vi "CAM_file_swap.vi"(8 "error in":errorcluster, 10 "DUT":string="1", 11 "Barcode":string) -> (0 "error out":errorcluster, 1 "Ref_img_path":path, 2 "DTU_Conf":string, 3 "image path":path)   [LabVIEW 2024, in "Keyence_VS150.lvlib"]
uses:
  Keyence_VS150.lvlib
  Launcher/Launcher_DTU.lvlib
panel:
  out "result string":string
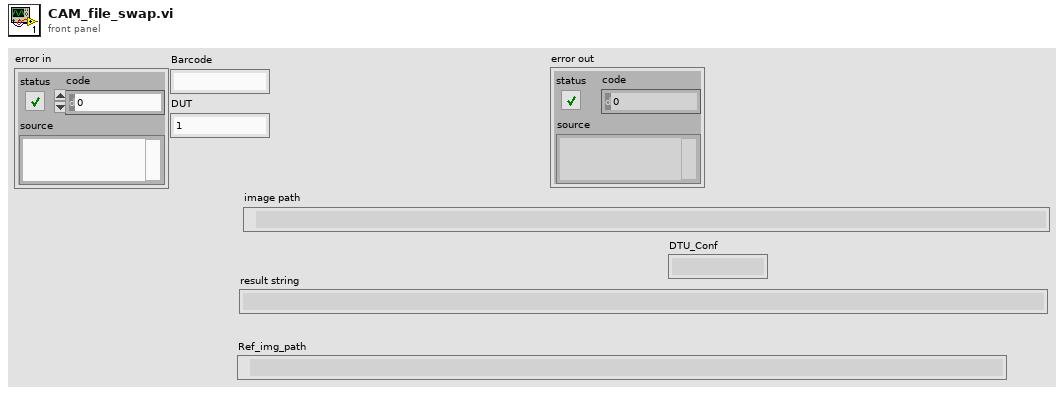
[diagram p1: front panel]
types:
  T1 = enum16{"Read", "Write", "All_sections", "All_values", "Remove key&section"}
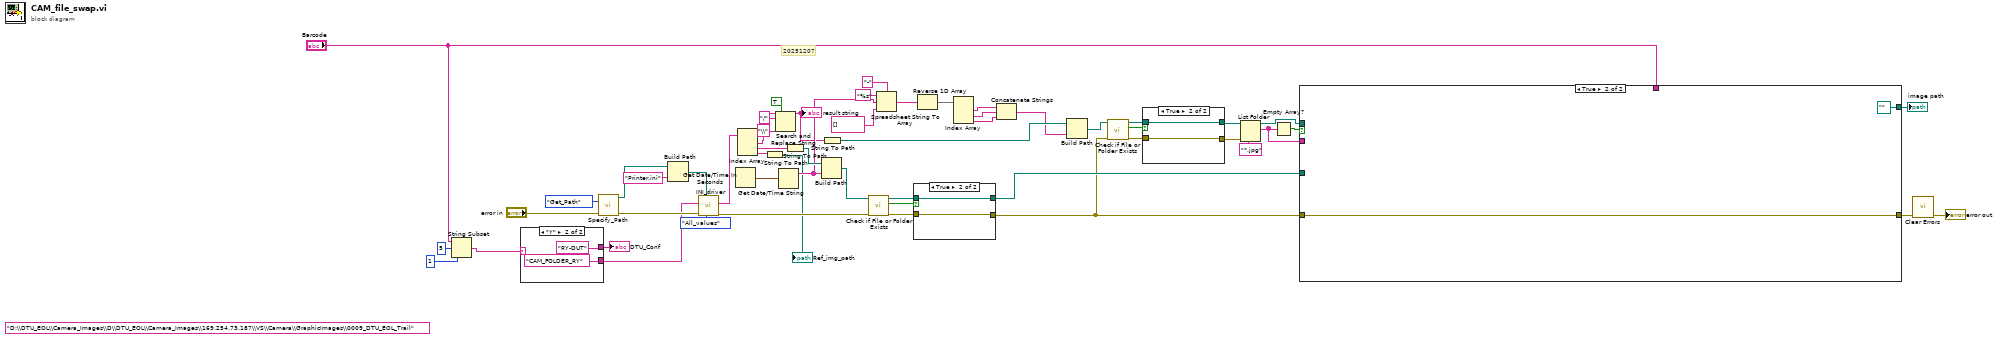
[diagram p0: block diagram]
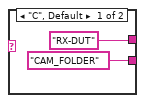
[diagram p2: hidden frame]
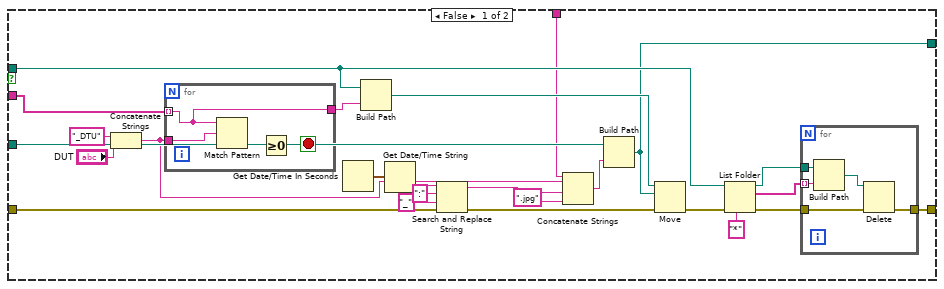
[diagram p3: hidden frame]
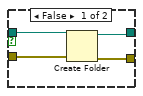
[diagram p4: hidden frame]
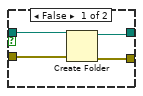
[diagram p5: hidden frame]
diagram:
  (unwired) "D:\\DTU_EOL\\Camera_Images\\D\\DTU_EOL\\Camera_Images\\169.254.73.187\\VS\\Camera\\GraphicImages\\0009_DTU_EOL_Trail"
  # "20251207"
  n1 = String Subset(string="Barcode", offset (0)=5, length (rest)=1 ("length (rest)")) -> (substring=w7:string)
  n2 = case shown="\"Y\"" w7 {
    tunnel: ["CAM_FOLDER" ("Section") "CAM_FOLDER_RY" ("Section")] -> w6
    tunnel: ["RX-DUT" "RY-DUT"] -> w3
    frame "C", Default {
    }
    frame "Y" {
    }
  }
  "DTU_Conf" <- w3
  n3 = call "Specify_Path.vi"("Path_Enum"=enum16{"Find_Path", "Get_Path"}."Get_Path", "error in (no error)"="error in") -> ("Configurations"=w52:path, "error out"=w53:errorcluster)  [unwired: 6 in, 6 out]
  n4 = Build Path(base path=w52, name or relative path="Printer.ini") -> (appended path=w50:path)
  n5 = call "INI_driver.vi"("Enum"=T1."All_values", "instrument file path"=w50, "error in (no error)"=w53, "Section"=w6) -> ("error out"=w45:errorcluster, "Values out"=w48:string[])  [unwired: 4 in, 2 out]
  n6 = Get Date/Time In Seconds() -> (seconds since 1Jan1904=w47:timestamp)
  n7 = Index Array(array=w48) -> (element #1=w14:string, element #2=w41:string, element #3=w2:string)  [unwired: 3 in]
  n8 = String To Path(string=w2) -> (path=→"Ref_img_path":path)
  n9 = Search and Replace String(replace all?=TRUE ("replace all? (F)"), input string=w14, search string="/", replace string="\\" ("replace string (\"\")")) -> (result string=w11:string)  [unwired: 4 in, 3 out]
  "result string" <- w11
  n10 = Get Date/Time String(seconds (now)=w47) -> (date string=w29:string)  [unwired: 2 in, 1 out]
  n11 = String To Path(string=w41) -> (path=w40:path)
  n12 = Build Path(base path=w40, name or relative path=w29) -> (appended path=w46:path)
  n13 = String To Path(string=w11) -> (path=w28:path)
  n14 = call <vilib>:"Check if File or Folder Exists.vi"("error in (no error)"=w45, "path"=w46) -> ("error out"=w42:errorcluster, "file or folder exists?"=w44:bool, "dup path"=w43:path)  [unwired: 7 in]
  n15 = Spreadsheet String To Array(delimiter (Tab)="-", format string="%s", spreadsheet string=w29, array type (2D Dbl)=string[] []) -> (array=w34:string[])
  n16 = case shown="True" w44 {
    tunnel: w43 -> [w62 w64]
    tunnel: w42 -> [w63 w65]
    tunnel: [w61 w65] -> w22
    tunnel: [w60 w64] -> w39
    frame False {
      n17 = Create Folder(path (use dialog)=w62, error in=w63) -> (created path=w60:path, error out=w61:errorcluster)  [unwired: 1 in, 1 out]
    }
    frame True {
    }
  }
  n18 = Reverse 1D Array(array=w34) -> (reversed array=w33:string[])
  n19 = Index Array(array=w33) -> (element #1=w32:string, element #2=w31:string, element #3=w30:string)  [unwired: 3 in]
  n20 = Concatenate Strings(w32, w31, w30) -> (w27:string)
  n21 = Build Path(base path=w28, name or relative path=w27) -> (appended path=w23:path)
  n22 = call <vilib>:"Check if File or Folder Exists.vi"("error in (no error)"=w22, "path"=w23) -> ("error out"=w26:errorcluster, "file or folder exists?"=w24:bool, "dup path"=w25:path)  [unwired: 7 in]
  n23 = case shown="True" w24 {
    tunnel: w25 -> [w68 w70]
    tunnel: w26 -> [w69 w71]
    tunnel: [w67 w71] -> w21
    tunnel: [w66 w70] -> w20
    frame False {
      n24 = Create Folder(path (use dialog)=w68, error in=w69) -> (created path=w66:path, error out=w67:errorcluster)  [unwired: 1 in, 1 out]
    }
    frame True {
    }
  }
  n25 = List Folder(path=w20, pattern="*.jpg", error in=w21) -> (path out=w17:path, filenames=w16:string[])  [unwired: 1 in, 2 out]
  n26 = Empty Array?(array=w16) -> (empty?=w18:bool)
  n27 = case shown="True" w18 {
    tunnel: w39 -> [w95 _]
    tunnel: [w78 w106] -> w38
    tunnel: w22 -> [w87 w106]
    tunnel: w17 -> [w74 _]
    tunnel: w16 -> [w84 _]
    tunnel: "Barcode" -> [w73 _]
    tunnel: [w72 path "" ("appended path")] -> w4
    frame False {
      n28 = Concatenate Strings("_DTU", "DUT") -> (w82:string)
      n29 = for {
        tunnel: w84 -> [w101] mode=indexing
        tunnel: w82 -> [w104]
        tunnel: [w101] -> w83
        stop <- w103 stop-if-true
        n30 = Match Pattern(string=w101, regular expression=w104) -> (offset past match=w102:i32)  [unwired: 1 in, 3 out]
        n31 = Greater Or Equal To 0?(x=w102) -> (x >= 0?=w103:bool)
      }
      n32 = Get Date/Time In Seconds() -> (seconds since 1Jan1904=w92:timestamp)
      n33 = Build Path(base path=w74, name or relative path=w83) -> (appended path=w81:path)
      n34 = Get Date/Time String(seconds (now)=w92) -> (time string=w91:string)  [unwired: 2 in, 1 out]
      n35 = Search and Replace String(input string=w91, search string=":", replace string="_" ("replace string (\"\")")) -> (result string=w88:string)  [unwired: 5 in, 3 out]
      n36 = Concatenate Strings(w73, w82, w88, ".jpg" ("string")) -> (w94:string)
      n37 = Build Path(base path=w95, name or relative path=w94) -> (appended path=w72:path)
      n38 = Move(source path=w81, error in=w87, 10:w72) -> (error out=w80:errorcluster)  [unwired: 2 in, 2 out]
      n39 = List Folder(path=w74, pattern="*", error in=w80) -> (path out=w77:path, filenames=w76:string[], error out=w79:errorcluster)  [unwired: 1 in, 1 out]
      n40 = for {
        tunnel: w77 -> [w98]
        tunnel: w79 -> [w100]
        tunnel: [w99] -> w78
        tunnel: w76 -> [w97] mode=indexing
        n41 = Build Path(base path=w98, name or relative path=w97) -> (appended path=w96:path)
        n42 = Delete(path (use dialog)=w96, error in=w100) -> (error out=w99:errorcluster)  [unwired: 3 in, 2 out]
      }
    }
    frame True {
    }
  }
  "image path" <- w4
  n43 = call <vilib>:"Clear Errors.vi"("error in (no error)"=w38) -> ("error out"=→"error out":errorcluster)  [unwired: 5 in, 1 out]
